vi "Host-ItchParser-TestHarness.vi"() -> ()   [LabVIEW 2016]
uses:
  <vilib>/rvi/interface/RandomDataEmulation/nirviRandomDataOpen.vi
  <vilib>/rvi/interface/RandomDataEmulation/nirviRandomDataDMAMethods.vi
  <vilib>/rvi/interface/RandomDataEmulation/nirviRandomDataClose.vi
  <vilib>/rvi/interface/nirviOpenFPGA/nirviOpenFPGA.xnode
  ItchParser-TestHarness-Typedef.ctl
  Fpga/Tests/Fpga-ItchParser-TestHarness.vi
  <vilib>/rvi/interface/nirviMethod/nirviMethod.xnode
  <vilib>/rvi/interface/nirviCloseFPGA/nirviCloseFPGA.xnode
panel:
  out "Timestamps":u64[](array[numeric])
  out "error out":errorcluster
  in  "file path (use dialog)":path
  in  "error in":errorcluster
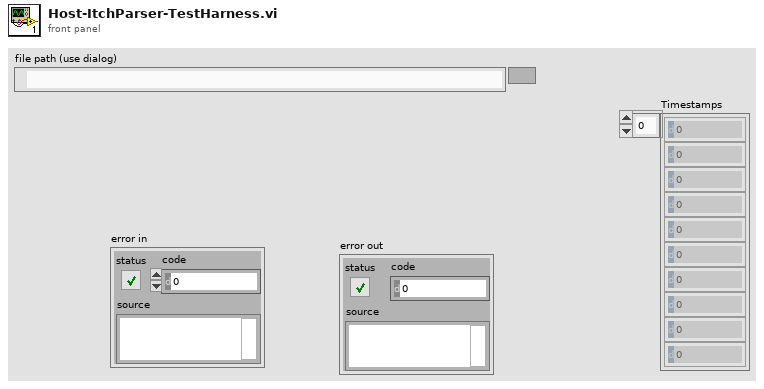
[diagram p1: front panel]
types:
  T1 = typedef "ItchParser-TestHarness-Typedef.ctl" = refnum<k20>
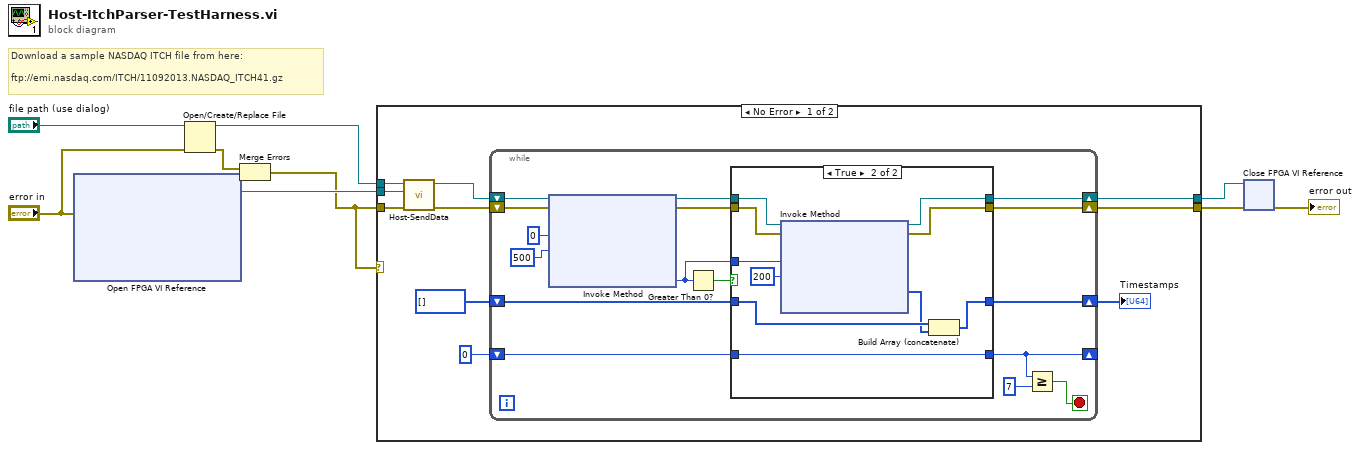
[diagram p0: block diagram]
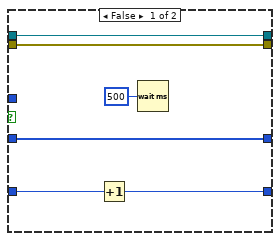
[diagram p2: hidden frame]
diagram:
  # "Download a sample NASDAQ ITCH file from here:\n\nftp://emi.nasdaq.com/ITCH/11092013.NASDAQ_ITCH41.gz"
  n1 = xnode "Open FPGA VI Reference"("error in"="error in") -> ("FPGA VI Reference Out"=w10:T1, "error out"=w5:errorcluster)  [unwired: 1 in]
  n2 = Open/Create/Replace File(file path (use dialog)="file path (use dialog)", error in="error in") -> (refnum out=w8:refnum<file>, error out=w6:errorcluster)  [unwired: 4 in, 1 out]
  n3 = Merge Errors(w6, w5) -> (w4:errorcluster)
  n4 = case shown="No Error" w4 {
    tunnel: w10 -> [w20 w53]
    tunnel: [w14 w54] -> w2
    tunnel: w8 -> [w17 _]
    tunnel: w4 -> [w15 w54]
    tunnel: [w13 w53] -> w1
    frame No Error {
      n5 = call "Host-SendData.vi"("error in\n(no error)"=w15, "FPGA VI Reference Out 3"=w20, "Byte Stream\nFile in"=w17) -> ("error out"=w18:errorcluster, "FPGA VI Reference Out 2"=w19:T1)  [unwired: 7 in]
      n6 = while {
        shift-right: [w25] -> w16
        shift-left: u64[] [] ("Data 2") -> [w26]
        shift-right: [w28] -> w13
        shift-left: w19 -> [w36]
        shift-right: [w27] -> w14
        shift-left: w18 -> [w29]
        shift-right: [w23] -> _
        shift-left: 0 -> [w24]
        stop <- w21 stop-if-true
        n7 = xnode "Invoke Method"("FPGA VI Reference In"=w36, "error in"=w29, "Number of Elements"=u32 0, "Timeout (ms)"=500) -> ("FPGA VI Reference Out"=w31:T1, "error out"=w30:errorcluster, "Elements Remaining"=w32:u32)  [unwired: 1 out]
        n8 = Greater Than 0?(x=w32) -> (x > 0?=w33:bool)
        n9 = case shown="True" w33 {
          tunnel: w32 -> [_ w52]
          tunnel: w31 -> [w42 w50]
          tunnel: w30 -> [w41 w49]
          tunnel: [w42 w48] -> w28
          tunnel: [w41 w47] -> w27
          tunnel: w26 -> [w40 w46]
          tunnel: [w40 w44] -> w25
          tunnel: [w38 w43] -> w23
          tunnel: w24 -> [w39 w43]
          frame False {
            n10 = Increment(x=w39) -> (x+1=w38:i32)
            n11 = Wait (ms)(milliseconds to wait=u32 500) -> ()  [unwired: 1 out]
          }
          frame True {
            n12 = xnode "Invoke Method"("FPGA VI Reference In"=w50, "error in"=w49, "Number of Elements"=w52, "Timeout (ms)"=200) -> ("FPGA VI Reference Out"=w48:T1, "error out"=w47:errorcluster, "Data"=w45:u64[])  [unwired: 1 out]
            n13 = Build Array (concatenate)(w46, w45) -> (w44:u64[])
          }
        }
        n14 = Greater Or Equal?(x=w23, y=7) -> (x >= y?=w21:bool)
      }
      "Timestamps" <- w16
    }
    frame Error {
    }
  }
  n15 = xnode "Close FPGA VI Reference"("FPGA VI Reference In"=w1, "error in"=w2) -> ("error out"=→"error out":errorcluster)
